vi "Kinesis - KBD101 - Set Velocity Parameters.vi"() -> ()   [LabVIEW 2012]
doc: "Shows how to set and get motor velocity parameters."
uses:
  U:/Kinesis LabVIEW Website Examples/Thorlabs.MotionControl.Controls.dll
  Thorlabs.MotionControl.Controls.dll
  U:/Kinesis LabVIEW Website Examples/Thorlabs.MotionControl.KCube.BrushlessMotorCLI.dll
  Thorlabs.MotionControl.KCube.BrushlessMotorCLI.dll
panel:
  out "Final VelParams":cluster{"maxVelocity":dbl, "acceleration":dbl}
  in  "Input VelParams":cluster{"maxVelocity":dbl, "acceleration":dbl}
  out "Initial VelParams":cluster{"maxVelocity":dbl, "acceleration":dbl}
  in  "SerialNumber":string
  in  "KCubeBrushlessControl":refnum<k24>(container)
  # "Notes:"
  # "- Ensure that the appropriate .DLLs are copied into your Project Folder. Check that the correct bit type are used depending on your version of LabVIEW\ni.e. 32-bit or 64-bit.\n\n\n\n\n\n\n\n\n\n\n\n\n\n\n- Open the example VI through the LabVIEW Project Explorer to correctly load the User Interface from Thorlabs.MotionControl.Controls.dll."
  # "Thorlabs Hardware: KBD101 - K-Cube Brushless DC Servo Motor Controller\nhttps://www.thorlabs.com/newgrouppage9.cfm?objectgroup_id=5698\n\nDescription: This VI will enable you to communicate with KBD101 to control DC Brushless Stages. The VI shows the current velocity parameters of the device and allows the user to change these settings outside of the UI.\n\nInstructions: \n1) Connect your KBD101 device to your PC & power the device, ensuring your stage/actutator is connected. For full device setup, the device product manual can be found on our website here:\n https://www.thorlabs.com/thorproduct.cfm?partnumber=KBD101\n2) Enter the device serial number below.\n3) Enter your required values for maxVelocity & acceleration.\n3) Click 'Run' in the LabVIEW Toolbar."
  # "Example Image of .NET Controller - VI opened via Project Explorer/ not opened via Project Explorer"
  # "VI Not Opened via Project Explorer"
  # "VI Opened via Project Explorer"
  # "- To explore the range of methods available, please visit the .NET API, included with your Kinesis software.\n\n- For tips on building your own VIs with Thorlabs Motion Control Hardware, please see our LabVIEW Guide here.\nhttps://www.thorlabs.com/newgrouppage9.cfm?objectgroup_id=10285"
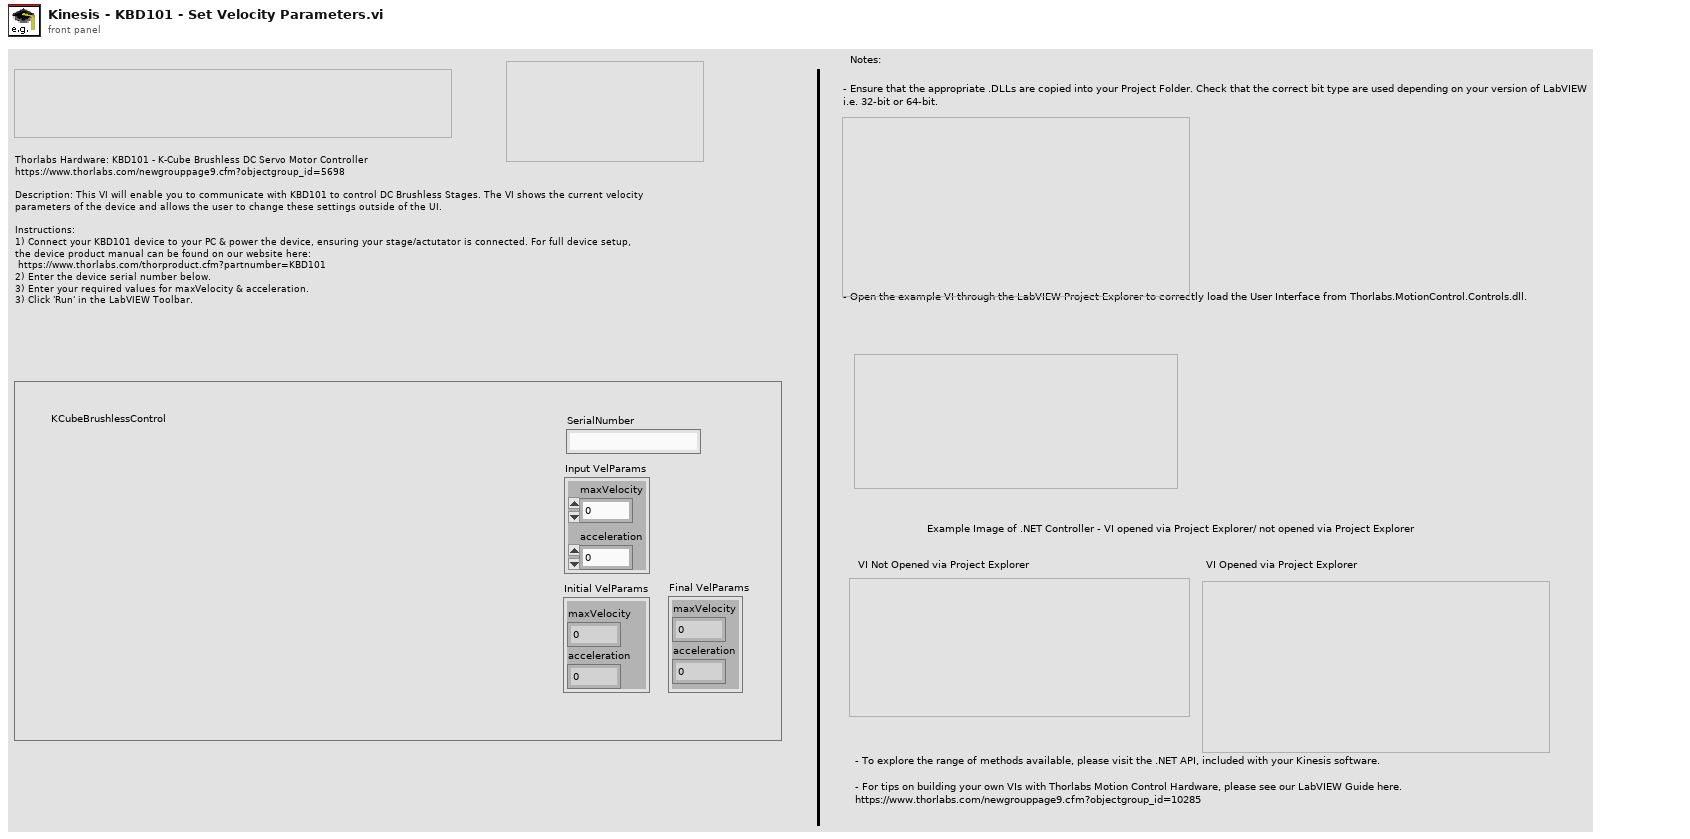
[diagram p1: front panel]
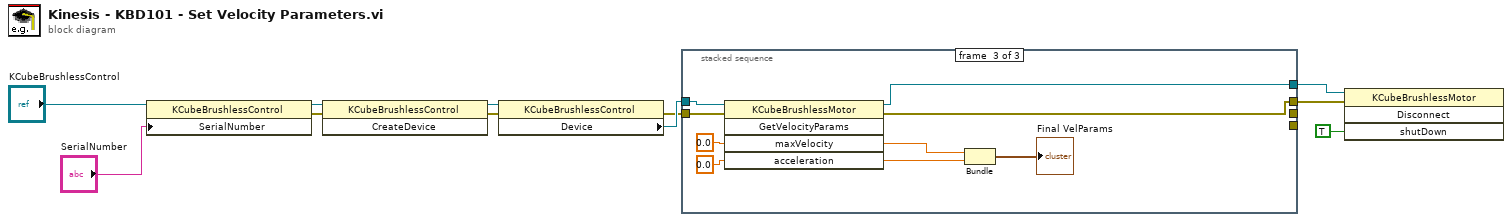
[diagram p0: block diagram]
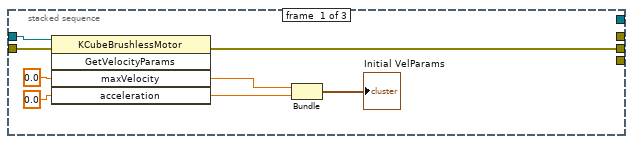
[diagram p2: hidden frame]
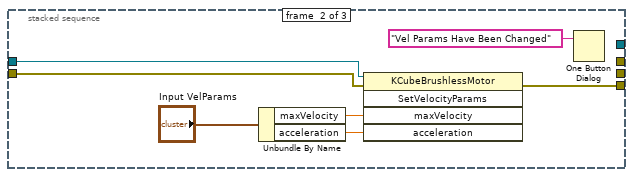
[diagram p3: hidden frame]
diagram:
  n1 = property class="KCubeBrushlessControl"(reference="KCubeBrushlessControl", "SerialNumber"="SerialNumber") -> (reference out=w8:refnum<k24>, error out=w6:errorcluster)  [unwired: 1 in]
  n2 = invoke class="KCubeBrushlessControl" method="CreateDevice"(reference=w8, error in=w6) -> (reference out=w7:refnum<k24>, error out=w5:errorcluster)  [unwired: 1 in, 1 out]
  n3 = property class="KCubeBrushlessControl"(reference=w7, error in=w5) -> (error out=w3:errorcluster, "Device"=w4:refnum<k24>)  [unwired: 1 out]
  n4 = stacked-sequence {
    tunnel: w4 -> [w19 w26 w29]
    tunnel: w3 -> [w16 w25 w30]
    tunnel: [w15 _ _] -> _
    tunnel: [_ w21 _] -> _
    tunnel: [_ _ w28] -> w2
    tunnel: [_ _ w27] -> w1
    frame #0 {
      n5 = invoke class="KCubeBrushlessMotor" method="GetVelocityParams"(reference=w19, error in=w16, "maxVelocity"=0.0, "acceleration"=0.0) -> (error out=w15:errorcluster, "maxVelocity"=w14:dbl, "acceleration"=w13:dbl)  [unwired: 1 in, 2 out]
      n6 = Bundle("maxVelocity"=w14, "acceleration"=w13) -> (→"Initial VelParams":cluster{"maxVelocity":dbl, "acceleration":dbl})  [unwired: 1 in]
    }
    frame #1 {
      n7 = Unbundle By Name("Input VelParams") -> ("maxVelocity"=w24:dbl, "acceleration"=w22:dbl)
      n8 = invoke class="KCubeBrushlessMotor" method="SetVelocityParams"(reference=w26, error in=w25, "maxVelocity"=w24, "acceleration"=w22) -> (error out=w21:errorcluster)  [unwired: 1 in, 4 out]
      n9 = One Button Dialog(message="Vel Params Have Been Changed") -> ()  [unwired: 1 in, 1 out]
    }
    frame #2 {
      n10 = invoke class="KCubeBrushlessMotor" method="GetVelocityParams"(reference=w29, error in=w30, "maxVelocity"=0.0, "acceleration"=0.0) -> (reference out=w27:refnum<k24>, error out=w28:errorcluster, "maxVelocity"=w33:dbl, "acceleration"=w32:dbl)  [unwired: 1 in, 1 out]
      n11 = Bundle("maxVelocity"=w33, "acceleration"=w32) -> (→"Final VelParams":cluster{"maxVelocity":dbl, "acceleration":dbl})  [unwired: 1 in]
    }
  }
  n12 = invoke class="KCubeBrushlessMotor" method="Disconnect"(reference=w1, error in=w2, "shutDown"=TRUE) -> ()  [unwired: 1 in, 4 out]
